vi "AggregatePulsePositions.vi"(8 "data flow maps":T1[](array[typedef]), 9 "new pulse positions array":T2[](array[typedef]), 10 "block count":i32, 11 "pulse positions array aggregate":T2[](array[typedef])) -> (3 "pulse positions array aggregate out":T2[](array[typedef]))   [LabVIEW 2017, in "CmsAcquisition.lvlib"]
uses:
  <vilib>/addons/InsightCM/Devices/Shared/Cms/CmsAcquisition/CmsAcquisition.lvlib
  <vilib>/addons/InsightCM/Utilities/Analysis/Shared/controls/PulsePositions.ctl
  <vilib>/addons/PointValueMap/controls/PointMap.ctl
  <vilib>/addons/PointValueMap/subVIs/Point_Read_double.vi
  <vilib>/addons/PointValueMap/PointValueMap.lvlib
  <vilib>/addons/InsightCM/Utilities/Analysis/Shared/AnalysisHelper.lvlib
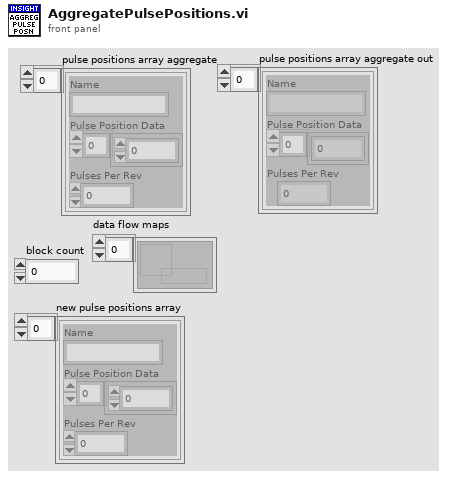
[diagram p1: front panel]
types:
  T1 = typedef "PointValueMap.lvlib/PointMap.ctl" = refnum<data-value>
  T2 = typedef "AnalysisHelper.lvlib/PulsePositions.ctl" = cluster{"Name":string, "Pulse Position Data":dbl[], "Pulses Per Rev":i32}
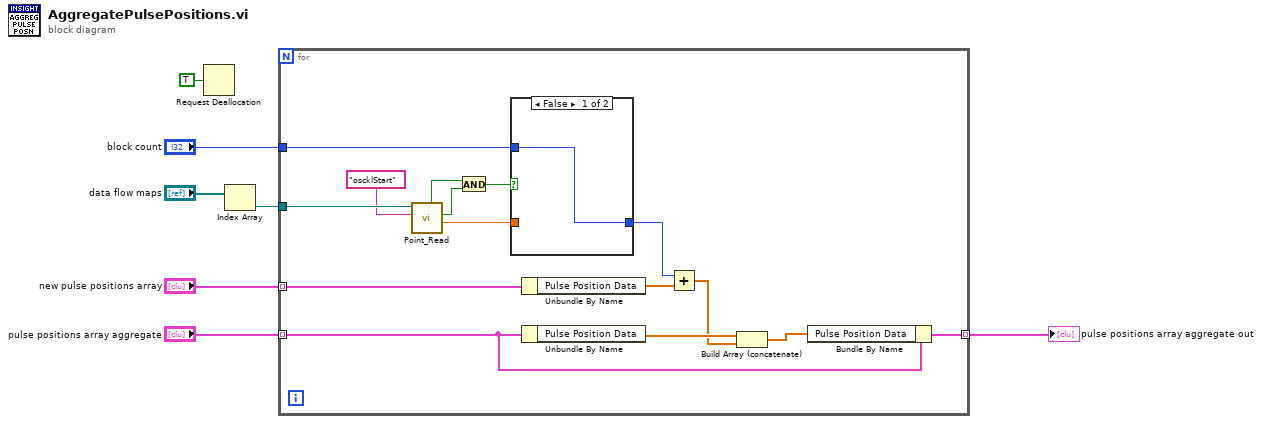
[diagram p0: block diagram]
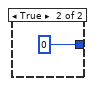
[diagram p2: hidden frame]
diagram:
  n1 = Request Deallocation(TRUE ("flag")) -> ()
  n2 = Index Array(array="data flow maps") -> (element=w2:T1)  [unwired: 1 in]
  n3 = for {
    tunnel: "new pulse positions array" -> [w22] mode=indexing
    tunnel: [w21] -> w6 mode=indexing
    tunnel: "pulse positions array aggregate" -> [w20] mode=indexing
    tunnel: "block count" -> [w19]
    tunnel: w2 -> [w18]
    n4 = call-poly <vilib>:"Point_Read.vi"("Tag"="oscklStart", "Map"=w18) -> ("Value"=w9:dbl, "Found?"=w17:bool, "Valid?"=w16:bool)  [unwired: 4 in, 3 out]
    n5 = And(x=w16, y=w17) -> (x .and. y?=w10:bool)
    n6 = case shown="False" w10 {
      tunnel: w9 -> [_ _]
      tunnel: [w23 0 ("block count")] -> w8
      tunnel: w19 -> [w23 _]
      frame False {
      }
      frame True {
      }
    }
    n7 = Unbundle By Name(w22) -> ("Pulse Position Data"=w12:dbl[])
    n8 = Unbundle By Name(w20) -> ("Pulse Position Data"=w14:dbl[])
    n9 = Add(x=w8, y=w12) -> (x+y=w11:dbl[])
    n10 = Build Array (concatenate)(w14, w11) -> (w13:dbl[])
    n11 = Bundle By Name(cluster=w20, "Pulse Position Data"=w13) -> (w21:T2)
  }
  "pulse positions array aggregate out" <- w6
